vi "Convert To Dev DTRow.vi"(8 "error in (no error)":errorcluster, 11 "DevInfo in":refnum<class "DevInfo.lvclass">) -> (0 "error out":errorcluster, 2 "Dev DTRow":string[](array[string])=["", "False", "False", "off.png", "", "Enter a label", "", "", ""], 3 "DevInfo out":refnum<class "DevInfo.lvclass">)   [LabVIEW 2016, in "Hardware.lvlib" / "DevInfo.lvclass"]
uses:
  <userlib>/Common Components/Hardware/DevInfo/DevInfo.lvclass
  <userlib>/Common Components/Hardware/DevInfo/DevInfo Cluster Constant.ctl
  <userlib>/Common Components/Hardware/DevInfo/DevInfo.lvclass/DevInfo.ctl
  <userlib>/Common Components/Hardware/DevInfo/Read GUID.vi
  <userlib>/Common Components/Hardware/DevInfo/Read Checked-out.vi
  <userlib>/Common Components/Hardware/DevInfo/Read Status.vi
  <userlib>/Common Components/Hardware/DevInfo/Read HW Type.vi
  <userlib>/Common Components/Hardware/DevInfo/Read Device Name.vi
  <userlib>/Common Components/Hardware/DevInfo/Read Label.vi
  <userlib>/Common Components/Hardware/DevInfo/Read COMM Address.vi
  <userlib>/Common Components/Hardware/DevInfo/Read Sub-COMM Address.vi
  <userlib>/Common Components/Hardware/DevInfo/Read COMM Settings.vi
  <userlib>/Common Components/Common/Common.lvlib
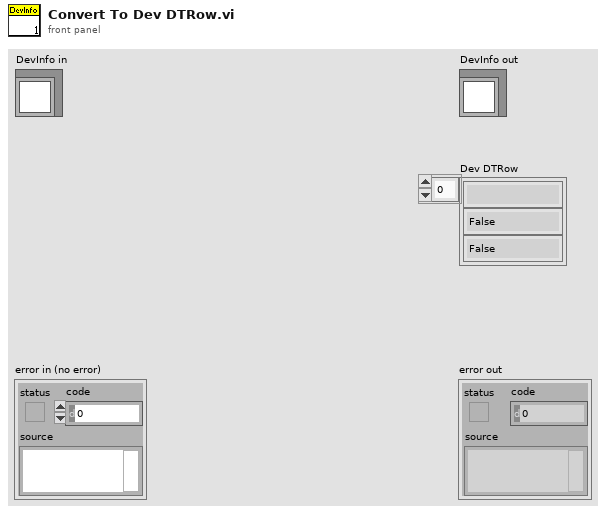
[diagram p1: front panel]
types:
  T1 = typedef "Hardware.lvlib/DevInfo.lvclass/DevInfo Cluster Constant.ctl" = cluster{"GUID":string, "Check":string, "Checked-out":string, "Status":string, "Device":string, "Label":string, "COMM":string, "Sub-COMM":string, "COMM Settings":string}
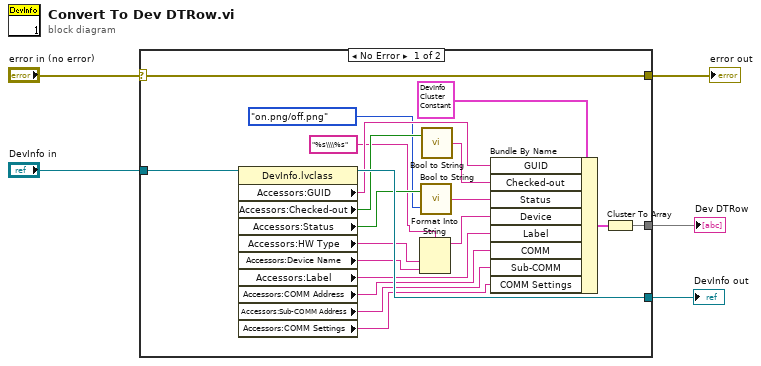
[diagram p0: block diagram]
diagram:
  n1 = case shown="No Error" "error in (no error)" {
    selector: "error in (no error)" -> [w24 w27]
    tunnel: [w24 w27] -> w4
    tunnel: [w22 w26] -> w2
    tunnel: "DevInfo in" -> [w25 w26]
    tunnel: [w13 _] -> w1
    frame No Error {
      n2 = property class="DevInfo.lvclass"(reference=w25) -> (reference out=w22:refnum<class "DevInfo.lvclass">, "Accessors:GUID"=w21:string, "Accessors:Checked-out"=w20:bool, "Accessors:Status"=w12:bool, "Accessors:HW Type"=w8:string, "Accessors:Device Name"=w7:string, "Accessors:Label"=w18:string, "Accessors:COMM Address"=w17:string, "Accessors:Sub-COMM Address"=w16:string, "Accessors:COMM Settings"=w15:string)  [unwired: 1 in, 1 out]
      n3 = Format Into String(format string="%s\\\\%s", w8, w7) -> (resulting string=w6:string)  [unwired: 2 in, 1 out]
      n4 = call <userlib>:"Bool to String.vi"("type (True/False)"=enum16{"True/False", "on.png/off.png"}."on.png/off.png" ("type"), "Boolean"=w12) -> ("Bool String"=w10:string)
      n5 = call <userlib>:"Bool to String.vi"("Boolean"=w20) -> ("Bool String"=w19:string)  [unwired: 1 in]
      n6 = Bundle By Name(cluster=T1 {"GUID"="", "Check"="False", "Checked-out"="False", "Status"="off.png", "Device"="", "Label"="Enter a label", "COMM"="", "Sub-COMM"="", "COMM Settings"=""} ("Cluster"), "GUID"=w21, "Checked-out"=w19, "Status"=w10, "Device"=w6, "Label"=w18, "COMM"=w17, "Sub-COMM"=w16, "COMM Settings"=w15) -> (w14:T1)
      n7 = Cluster To Array(cluster=w14) -> (array=w13:string[])
    }
    frame Error {
    }
  }
  "error out" <- w4
  "DevInfo out" <- w2
  "Dev DTRow" <- w1
